vi "Piezo_Positioning_MD.vi"() -> ()   [LabVIEW 2012]
uses:
  <vilib>/DAQmx/write.llb/DAQmx Write (Analog DBL 1Chan 1Samp).vi
  GFG/GFGbooleanGet.vi
  <vilib>/DAQmx/create/channels.llb/DAQmx Create Channel (AO-Voltage-Basic).vi
  <vilib>/DAQmx/miscellaneous.llb/DAQmx Fill In Error Info.vi
  GFG/GFGnumericGet.vi
  GFG/GFG library.lvlib
panel:
  in  "Step Size (um)":u16(ring)=5 items=["1"=1, "2"=2, "5"=5, "10"=10, "20"=20, "50"=50, "100"=100]
  in  "Z DOWN":bool
  in  "Z UP":bool
  in  "Z-Spacing (microns)":dbl=1.0 min=0.1
  in  "Clear Stack":bool
  in  "Remove Last":bool
  in  "Add Plane":bool
  out "Configured Stack":dbl[][](array[numeric])
  in  "Z - Piezo Offset  (um)":i32 max=600
  # "X"
  # "Y"
  # "Z"
  # "Laser 1"
  # "Laser 2"
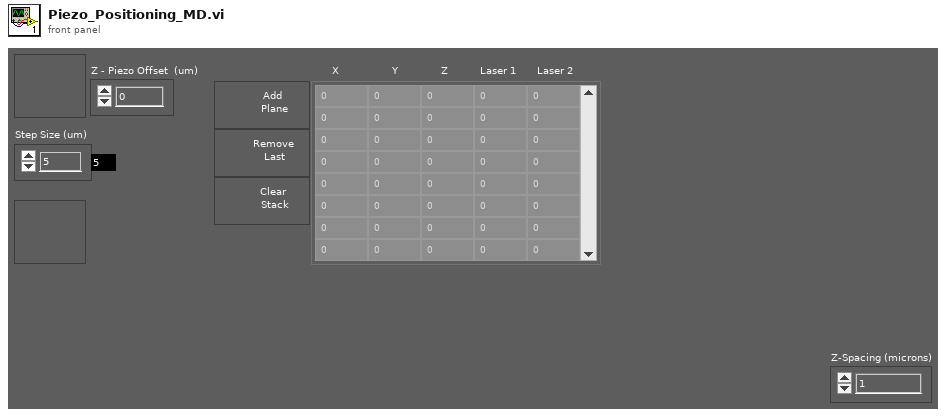
[diagram p1: front panel]
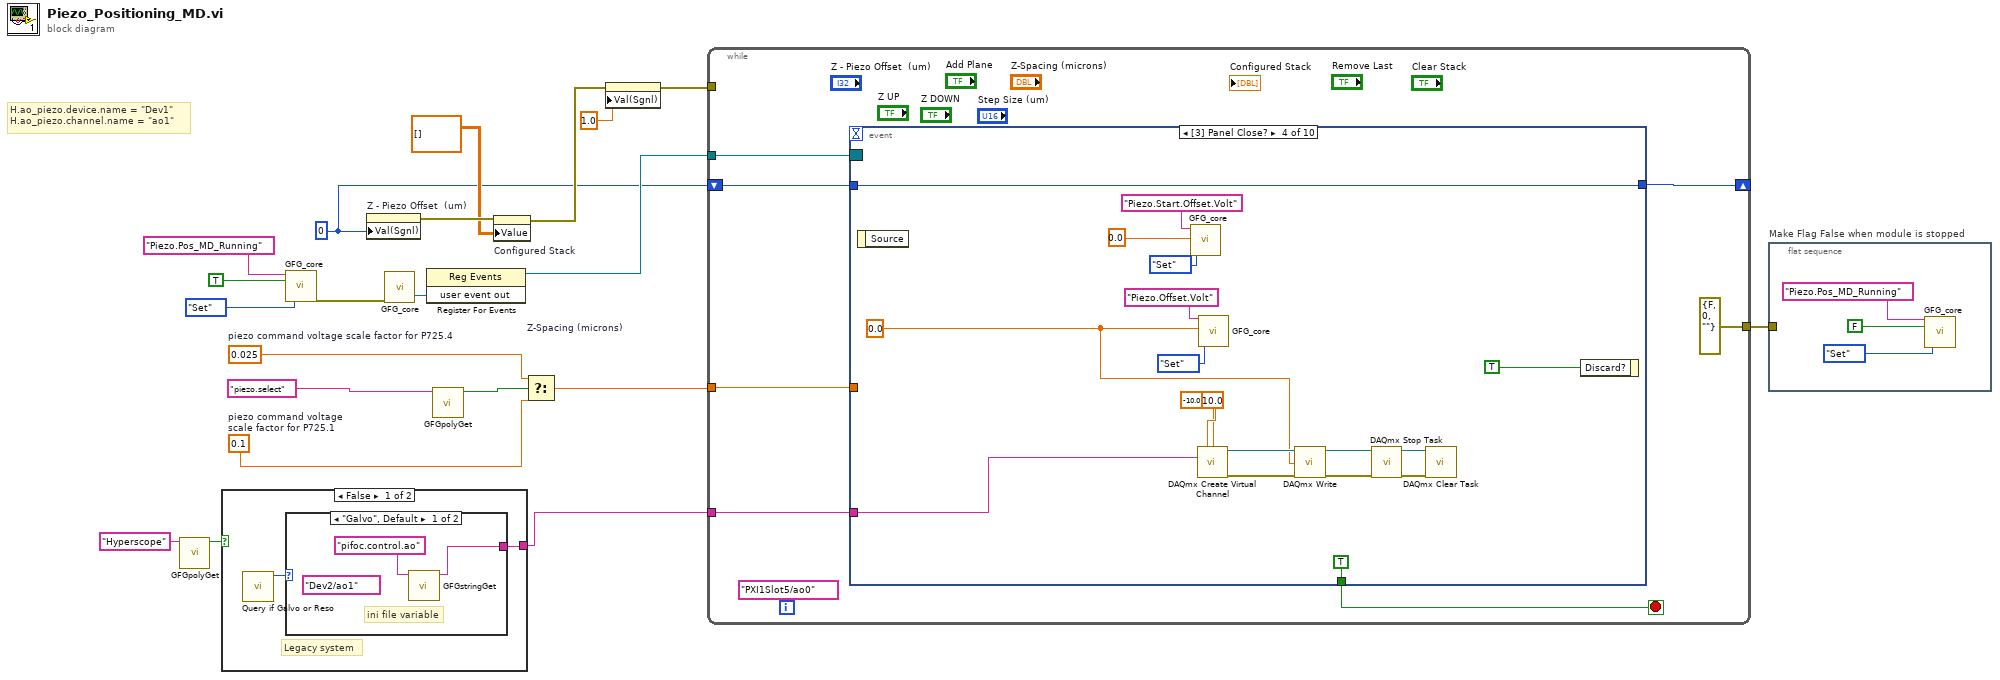
[diagram p0: block diagram]
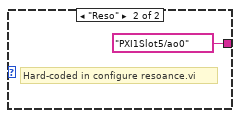
[diagram p2: hidden frame]
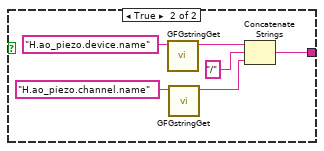
[diagram p3: hidden frame]
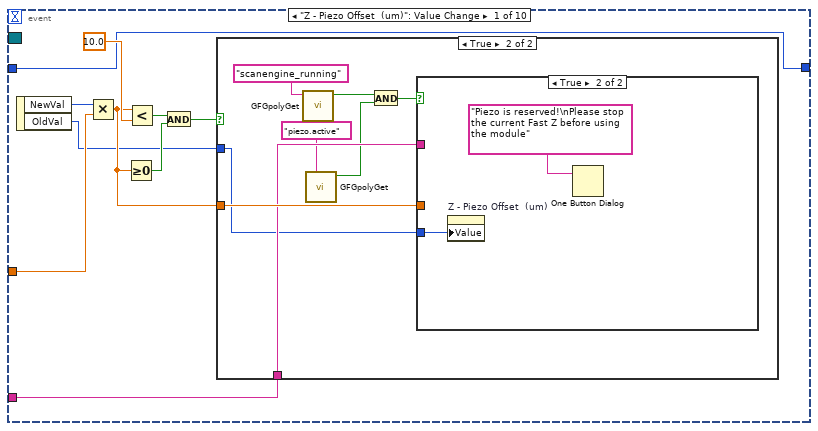
[diagram p4: hidden frame]
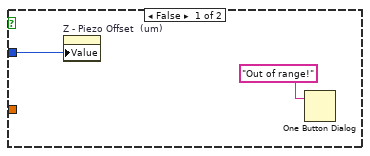
[diagram p5: hidden frame]
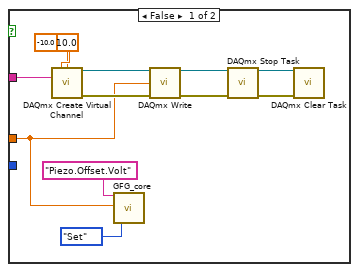
[diagram p6: hidden frame]
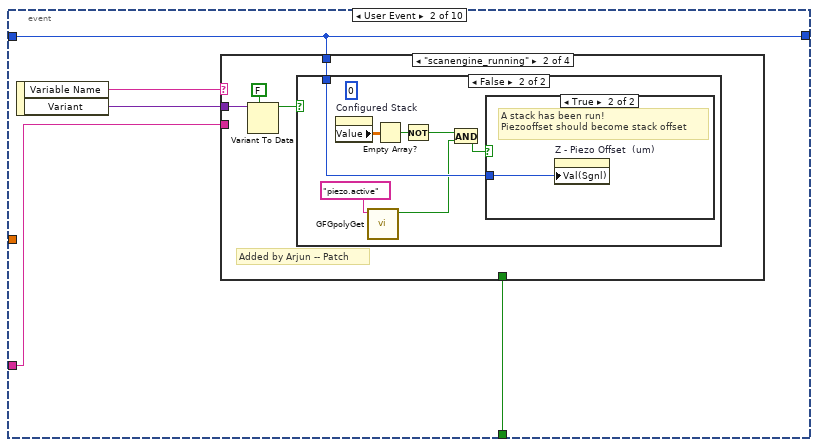
[diagram p7: hidden frame]
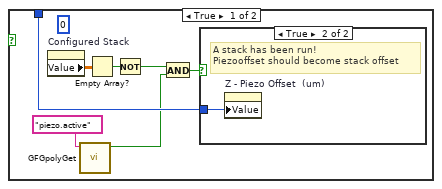
[diagram p9: hidden frame]
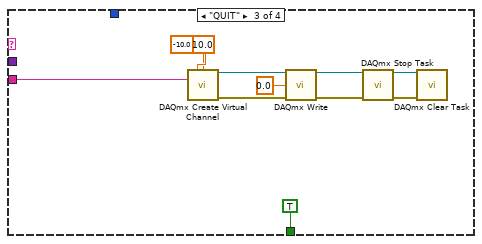
[diagram p12: hidden frame]
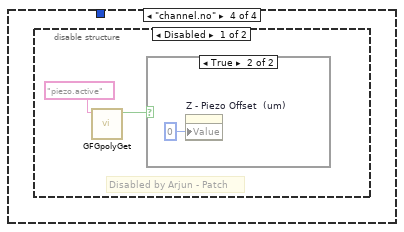
[diagram p13: hidden frame]
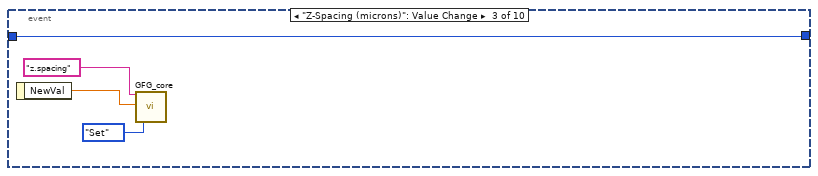
[diagram p16: hidden frame]
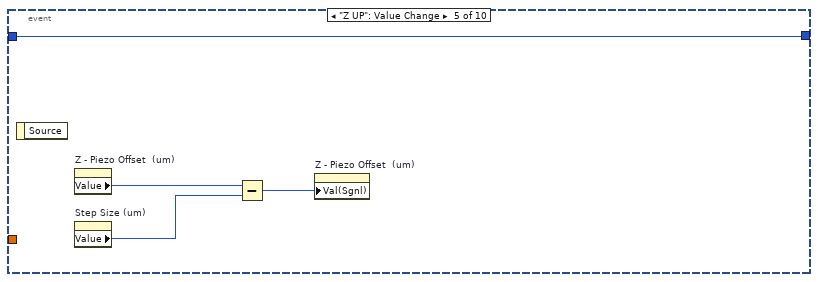
[diagram p17: hidden frame]
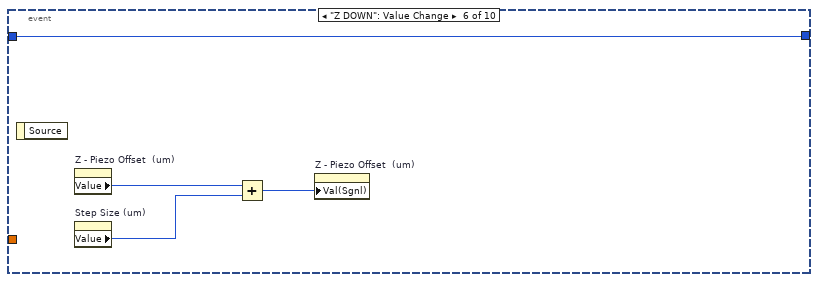
[diagram p18: hidden frame]
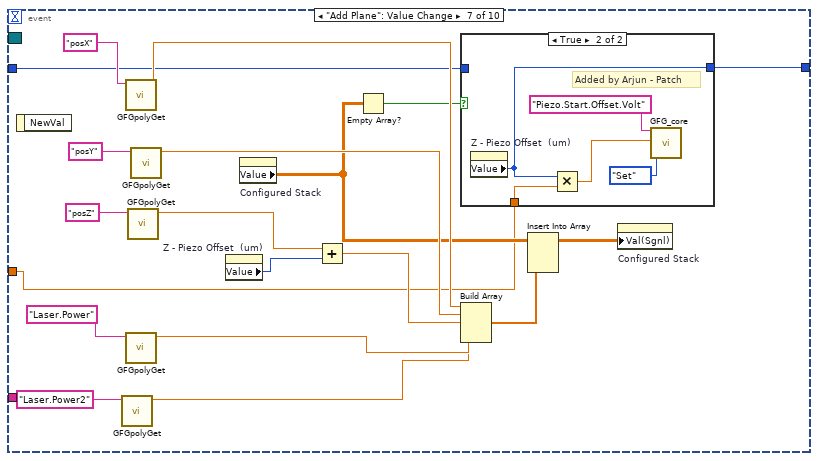
[diagram p19: hidden frame]
diagram:
  w9 = 0 ("Value (Signaling)")
  w18 = 0.1  # piezo command voltage scale factor for P725.1
  w19 = 0.025  # piezo command voltage scale factor for P725.4
  # "H.ao_piezo.device.name = \"Dev1\"\nH.ao_piezo.channel.name = \"ao1\""
  n1 = call-poly "GFGpolyGet.vi"("Variable Name in"="Hyperscope") -> ("Boolean Value OUT"=w2:bool)  [unwired: 9 in, 1 out]
  n2 = case shown="False" w2 {
    tunnel: [w23 w27] -> w1
    frame False {
      # "Legacy system"
      n3 = call "Query if Galvo or Reso.vi"() -> ("System Type"=w22:enum16{"Galvo", "Reso"})  [unwired: 10 in, 1 out]
      n4 = case shown="\"Galvo\", Default" w22 {
        tunnel: [w24 tag "PXI1Slot5/ao0" ("AO Channel for Piezo")] -> w23
        frame "Galvo", Default {
          (unwired) tag "Dev2/ao1" ("AO Channel for Piezo")
          # "ini file variable"
          n5 = call "GFGstringGet.vi"("Variable Name in"="pifoc.control.ao") -> ("String"=w24:string)  [unwired: 9 in, 1 out]
        }
        frame "Reso" {
          # "Hard-coded in configure resoance.vi"
        }
      }
    }
    frame True {
      n6 = call "GFGstringGet.vi"("Variable Name in"="H.ao_piezo.device.name") -> ("String"=w30:string)  [unwired: 9 in, 1 out]
      n7 = call "GFGstringGet.vi"("Variable Name in"="H.ao_piezo.channel.name") -> ("String"=w28:string)  [unwired: 9 in, 1 out]
      n8 = Concatenate Strings(w30, "/" ("string"), w28) -> (w27:string)
    }
  }
  n9 = call "GFG_core.vi"("Variable Name in"="Piezo.Pos_MD_Running", "Variant in"=TRUE, "Action"=enum16{"Init", "Set", "Get", "Clear"}."Set") -> ("error out"=w5:errorcluster)  [unwired: 10 in, 6 out]
  n10 = property on="Z - Piezo Offset  (um)" class="DigNum (strict)"("Val(Sgnl)"=w9) -> (error out=w14:errorcluster)  [unwired: 2 in, 1 out]
  n11 = call "GFG_core.vi"("error in (no error)"=w5) -> ("user event out"=w11:refnum<user-event>)  [unwired: 12 in, 6 out]
  n12 = register-events(w11) -> (reference out=w10:refnum<event-registration>)  [unwired: 2 in, 1 out]
  n13 = call-poly "GFGpolyGet.vi"("Variable Name in"="piezo.select") -> ("Boolean Value OUT"=w16:bool)  [unwired: 9 in, 1 out]
  n14 = property on="Configured Stack" class="Arr (strict)"(error in=w14, "Value"=dbl[][] []) -> (error out=w12:errorcluster)  [unwired: 1 in, 1 out]
  n15 = Select(t=w19, s=w16, f=w18) -> (s? t:f=w15:dbl)
  n16 = property on="Z-Spacing (microns)" class="DigNum (strict)"(error in=w12, "Val(Sgnl)"=1.0 ("Value (Signaling)")) -> (error out=w20:errorcluster)  [unwired: 1 in, 1 out]
  n17 = while {
    tunnel: w20 -> [_]
    tunnel: w15 -> [w38]
    tunnel: w10 -> [w37]
    shift-right: [w36] -> _
    shift-left: w9 -> [w35]
    tunnel: [errorcluster {"status"=FALSE, "code"=0, "source"=""} ("error constant")] -> w4
    tunnel: w1 -> [w33]
    stop <- w39 stop-if-true
    (unwired) tag "PXI1Slot5/ao0" ("AO Channel for Piezo")
    n18 = event shown="[3] Panel Close?" {
      selector: w37 -> [_ _ _ _ _ _ _ _ _ _]
      dyn-events: _ -> [_ _ _ _ _ _ _ _ _ _]
      timeout: _ -> [_ _ _ _ _ _ _ _ _ _]
      tunnel: [_ w77 _ TRUE _ _ _ _ _ _] -> w39
      tunnel: w38 -> [w44 _ _ _ _ _ w145 w170 w184 _]
      tunnel: w33 -> [w41 w75 _ w119 _ _ _ _ _ _]
      tunnel: [w40 w74 w113 w117 w135 w139 w144 w168 w181 w191] -> w36
      tunnel: w35 -> [w40 w74 w113 w117 w135 w139 w143 w169 _ w191]
      event "Z - Piezo Offset  (um)": Value Change {
        n19 = event-data() -> ("NewVal"=w49:i32, "OldVal"=w42:i32)  [unwired: 1 in]
        n20 = Multiply(x=w49, y=w44) -> (x*y=w43:dbl)
        n21 = Greater Or Equal To 0?(x=w43) -> (x >= 0?=w45:bool)
        n22 = Less?(x=w43, y=10.0) -> (x < y?=w48:bool)
        n23 = And(x=w48, y=w45) -> (x .and. y?=w46:bool)
        n24 = case shown="True" w46 {
          tunnel: w43 -> [_ w59]
          tunnel: w42 -> [w50 w52]
          tunnel: w41 -> [_ w58]
          frame False {
            n25 = property on="Z - Piezo Offset  (um)" class="DigNum (strict)"("Value"=w50) -> ()  [unwired: 2 in, 2 out]
            n26 = One Button Dialog(message="Out of range!") -> ()  [unwired: 1 in, 1 out]
          }
          frame True {
            n27 = call-poly "GFGpolyGet.vi"("Variable Name in"="scanengine_running") -> ("Boolean Value OUT"=w55:bool)  [unwired: 9 in, 1 out]
            n28 = call-poly "GFGpolyGet.vi"("Variable Name in"="piezo.active") -> ("Boolean Value OUT"=w54:bool)  [unwired: 9 in, 1 out]
            n29 = And(x=w55, y=w54) -> (x .and. y?=w53:bool)
            n30 = case shown="True" w53 {
              tunnel: w59 -> [w61 _]
              tunnel: w58 -> [w60 _]
              tunnel: w52 -> [_ w72]
              frame False {
                n31 = call-poly <vilib>:"DAQmx Create Virtual Channel.vi"("maximum value"=10.0, "minimum value"=-10.0, "physical channels"=w60) -> ("task out"=w69:refnum<k21>, "error out"=w65:errorcluster)  [unwired: 11 in]
                n32 = call "GFG_core.vi"("Variable Name in"="Piezo.Offset.Volt", "Variant in"=w61, "Action"=enum16{"Init", "Set", "Get", "Clear"}."Set") -> ()  [unwired: 10 in, 7 out]
                n33 = call-poly <vilib>:"DAQmx Write.vi"("task/channels in"=w69, "data"=w61, "error in"=w65) -> ("task out"=w66:refnum<k21>, "error out"=w64:errorcluster)  [unwired: 10 in, 1 out]
                n34 = call <vilib>:"DAQmx Stop Task.vi"("task/channels in"=w66, "error in"=w64) -> ("task out"=w67:refnum<k21>, "error out"=w68:errorcluster)  [unwired: 12 in]
                n35 = call <vilib>:"DAQmx Clear Task.vi"("task in"=w67, "error in"=w68) -> ()  [unwired: 13 in, 1 out]
              }
              frame True {
                n36 = property on="Z - Piezo Offset  (um)" class="DigNum (strict)"("Value"=w72) -> ()  [unwired: 2 in, 2 out]
                n37 = One Button Dialog(message="Piezo is reserved!\nPlease stop the current Fast Z before using the module") -> ()  [unwired: 1 in, 1 out]
              }
            }
          }
        }
      }
      event User Event {
        n38 = event-data() -> ("Variable Name"=w78:string, "Variant"=w76:variant)  [unwired: 1 in]
        n39 = case shown="\"scanengine_running\"" w78 {
          tunnel: [_ _ TRUE _] -> w77
          tunnel: w76 -> [_ w82 _ _]
          tunnel: w75 -> [_ _ w100 _]
          tunnel: w74 -> [_ w79 _ _]
          frame "False", Default {
          }
          frame "scanengine_running" {
            # "Added by Arjun -- Patch"
            n40 = Variant To Data(type=FALSE, Variant=w82) -> (data=w80:bool)  [unwired: 1 in, 1 out]
            n41 = case shown="False" w80 {
              tunnel: w79 -> [w89 w97]
              frame True {
                (unwired) 0 ("Z - Piezo Offset  (um)")
                n42 = property on="Configured Stack" class="Arr (strict)"() -> ("Value"=w88:dbl[][])  [unwired: 2 in, 2 out]
                n43 = call-poly "GFGpolyGet.vi"("Variable Name in"="piezo.active") -> ("Boolean Value OUT"=w84:bool)  [unwired: 9 in, 1 out]
                n44 = Empty Array?(array=w88) -> (empty?=w87:bool)
                n45 = Not(x=w87) -> (.not. x?=w83:bool)
                n46 = And(x=w83, y=w84) -> (x .and. y?=w85:bool)
                n47 = case shown="True" w85 {
                  tunnel: w89 -> [_ w90]
                  frame False {
                  }
                  frame True {
                    # "A stack has been run!\nPiezooffset should become stack offset"
                    n48 = property on="Z - Piezo Offset  (um)" class="DigNum (strict)"("Value"=w90) -> ()  [unwired: 2 in, 2 out]
                  }
                }
              }
              frame False {
                (unwired) 0 ("Z - Piezo Offset  (um)")
                n49 = property on="Configured Stack" class="Arr (strict)"() -> ("Value"=w96:dbl[][])  [unwired: 2 in, 2 out]
                n50 = call-poly "GFGpolyGet.vi"("Variable Name in"="piezo.active") -> ("Boolean Value OUT"=w93:bool)  [unwired: 9 in, 1 out]
                n51 = Empty Array?(array=w96) -> (empty?=w95:bool)
                n52 = Not(x=w95) -> (.not. x?=w92:bool)
                n53 = And(x=w92, y=w93) -> (x .and. y?=w91:bool)
                n54 = case shown="True" w91 {
                  tunnel: w97 -> [_ w98]
                  frame False {
                  }
                  frame True {
                    # "A stack has been run!\nPiezooffset should become stack offset"
                    n55 = property on="Z - Piezo Offset  (um)" class="DigNum (strict)"("Val(Sgnl)"=w98) -> ()  [unwired: 2 in, 2 out]
                  }
                }
              }
            }
          }
          frame "QUIT" {
            n56 = call-poly <vilib>:"DAQmx Create Virtual Channel.vi"("maximum value"=10.0, "minimum value"=-10.0, "physical channels"=w100) -> ("task out"=w106:refnum<k21>, "error out"=w102:errorcluster)  [unwired: 11 in]
            n57 = call-poly <vilib>:"DAQmx Write.vi"("task/channels in"=w106, "data"=0.0 ("maximum value"), "error in"=w102) -> ("task out"=w103:refnum<k21>, "error out"=w101:errorcluster)  [unwired: 10 in, 1 out]
            n58 = call <vilib>:"DAQmx Stop Task.vi"("task/channels in"=w103, "error in"=w101) -> ("task out"=w104:refnum<k21>, "error out"=w105:errorcluster)  [unwired: 12 in]
            n59 = call <vilib>:"DAQmx Clear Task.vi"("task in"=w104, "error in"=w105) -> ()  [unwired: 13 in, 1 out]
          }
          frame "channel.no" {
            n60 = disable-structure shown="Disabled" {
              frame Disabled {
                # "Disabled by Arjun - Patch"
                n61 = call-poly "GFGpolyGet.vi"("Variable Name in"="piezo.active") -> ("Boolean Value OUT"=w110:bool)  [unwired: 9 in, 1 out]
                n62 = case shown="True" w110 {
                  frame False {
                  }
                  frame True {
                    n63 = property on="Z - Piezo Offset  (um)" class="DigNum (strict)"("Value"=0 ("Z - Piezo Offset  (um)")) -> ()  [unwired: 2 in, 2 out]
                  }
                }
              }
              frame Enabled {
              }
            }
          }
        }
      }
      event "Z-Spacing (microns)": Value Change {
        n64 = event-data() -> ("NewVal"=w114:dbl)  [unwired: 1 in]
        n65 = call "GFG_core.vi"("Variable Name in"="z.spacing", "Variant in"=w114, "Action"=enum16{"Init", "Set", "Get", "Clear"}."Set") -> ()  [unwired: 10 in, 7 out]
      }
      event Panel Close? {
        w118 = 0.0 ("Value (Signaling)")
        n66 = event-data() -> ()  [unwired: 1 in, 1 out]
        n67 = call "GFG_core.vi"("Variable Name in"="Piezo.Start.Offset.Volt", "Variant in"=0.0 ("Value (Signaling)"), "Action"=enum16{"Init", "Set", "Get", "Clear"}."Set") -> ()  [unwired: 10 in, 7 out]
        n68 = call-poly <vilib>:"DAQmx Create Virtual Channel.vi"("maximum value"=10.0, "minimum value"=-10.0, "physical channels"=w119) -> ("task out"=w125:refnum<k21>, "error out"=w121:errorcluster)  [unwired: 11 in]
        n69 = call "GFG_core.vi"("Variable Name in"="Piezo.Offset.Volt", "Variant in"=w118, "Action"=enum16{"Init", "Set", "Get", "Clear"}."Set") -> ()  [unwired: 10 in, 7 out]
        n70 = call-poly <vilib>:"DAQmx Write.vi"("task/channels in"=w125, "data"=w118, "error in"=w121) -> ("task out"=w122:refnum<k21>, "error out"=w120:errorcluster)  [unwired: 10 in, 1 out]
        n71 = call <vilib>:"DAQmx Stop Task.vi"("task/channels in"=w122, "error in"=w120) -> ("task out"=w123:refnum<k21>, "error out"=w124:errorcluster)  [unwired: 12 in]
        n72 = call <vilib>:"DAQmx Clear Task.vi"("task in"=w123, "error in"=w124) -> ()  [unwired: 13 in, 1 out]
        n73 = event-data("Discard?"=TRUE) -> ()  [unwired: 1 in, 1 out]
      }
      event "Z UP": Value Change {
        n74 = event-data() -> ()  [unwired: 1 in, 1 out]
        n75 = property on="Z - Piezo Offset  (um)" class="DigNum (strict)"() -> ("Value"=w138:i32)  [unwired: 2 in, 2 out]
        n76 = property on="Step Size (um)" class="Ring (strict)"() -> ("Value"=w137:u16)  [unwired: 2 in, 2 out]
        n77 = Subtract(x=w138, y=w137) -> (x-y=w136:i32)
        n78 = property on="Z - Piezo Offset  (um)" class="DigNum (strict)"("Val(Sgnl)"=w136) -> ()  [unwired: 2 in, 2 out]
      }
      event "Z DOWN": Value Change {
        n79 = event-data() -> ()  [unwired: 1 in, 1 out]
        n80 = property on="Z - Piezo Offset  (um)" class="DigNum (strict)"() -> ("Value"=w142:i32)  [unwired: 2 in, 2 out]
        n81 = property on="Step Size (um)" class="Ring (strict)"() -> ("Value"=w141:u16)  [unwired: 2 in, 2 out]
        n82 = Add(x=w142, y=w141) -> (x+y=w140:i32)
        n83 = property on="Z - Piezo Offset  (um)" class="DigNum (strict)"("Val(Sgnl)"=w140) -> ()  [unwired: 2 in, 2 out]
      }
      event "Add Plane": Value Change {
        n84 = event-data() -> ()  [unwired: 1 in, 1 out]
        n85 = call-poly "GFGpolyGet.vi"("Variable Name in"="Laser.Power2") -> ("Numeric"=w149:dbl)  [unwired: 8 in, 2 out]
        n86 = call-poly "GFGpolyGet.vi"("Variable Name in"="posX") -> ("Numeric"=w156:dbl)  [unwired: 8 in, 2 out]
        n87 = call-poly "GFGpolyGet.vi"("Variable Name in"="Laser.Power") -> ("Numeric"=w150:dbl)  [unwired: 8 in, 2 out]
        n88 = call-poly "GFGpolyGet.vi"("Variable Name in"="posZ") -> ("Numeric"=w157:dbl)  [unwired: 8 in, 2 out]
        n89 = call-poly "GFGpolyGet.vi"("Variable Name in"="posY") -> ("Numeric"=w155:dbl)  [unwired: 8 in, 2 out]
        n90 = property on="Z - Piezo Offset  (um)" class="DigNum (strict)"() -> ("Value"=w158:i32)  [unwired: 2 in, 2 out]
        n91 = property on="Configured Stack" class="Arr (strict)"() -> ("Value"=w147:dbl[][])  [unwired: 2 in, 2 out]
        n92 = Add(x=w157, y=w158) -> (x+y=w154:dbl)
        n93 = Empty Array?(array=w147) -> (empty?=w146:bool)
        n94 = case shown="True" w146 {
          tunnel: w145 -> [_ w165]
          tunnel: [w162 w163] -> w144
          tunnel: w143 -> [w162 _]
          frame False {
          }
          frame True {
            # "Added by Arjun - Patch"
            n95 = property on="Z - Piezo Offset  (um)" class="DigNum (strict)"() -> ("Value"=w163:i32)  [unwired: 2 in, 2 out]
            n96 = Multiply(x=w163, y=w165) -> (x*y=w164:dbl)
            n97 = call "GFG_core.vi"("Variable Name in"="Piezo.Start.Offset.Volt", "Variant in"=w164, "Action"=enum16{"Init", "Set", "Get", "Clear"}."Set") -> ()  [unwired: 10 in, 7 out]
          }
        }
        n98 = Build Array(w156, w155, w154, w150, w149) -> (w153:dbl[])
        n99 = Insert Into Array(array=w147, new element=w153) -> (w148:dbl[][])  [unwired: 2 in]
        n100 = property on="Configured Stack" class="Arr (strict)"("Val(Sgnl)"=w148) -> ()  [unwired: 2 in, 2 out]
      }
      event "Remove Last": Value Change {
        n101 = event-data() -> ()  [unwired: 1 in, 1 out]
        n102 = property on="Configured Stack" class="Arr (strict)"() -> ("Value"=w171:dbl[][])  [unwired: 2 in, 2 out]
        n103 = Empty Array?(array=w171) -> (empty?=w172:bool)
        n104 = case shown="True" w172 {
          tunnel: w170 -> [_ w176]
          tunnel: w169 -> [w174 _]
          tunnel: [w174 w175] -> w168
          frame False {
          }
          frame True {
            w178 = 0.0  # Stack start voltage
            # "Added by Arjun - Patch"
            n105 = Divide(x=w178, y=w176) -> (x/y=w177:dbl)
            n106 = To Long Integer(number=w177) -> (32bit integer=w175:i32)
            n107 = call "GFG_core.vi"("Variable Name in"="Piezo.Start.Offset.Volt", "Variant in"=w178, "Action"=enum16{"Init", "Set", "Get", "Clear"}."Set") -> ()  [unwired: 10 in, 7 out]
          }
        }
        n108 = Delete From Array(array=w171) -> (array with subset deleted=w173:dbl[][])  [unwired: 3 in, 1 out]
        n109 = property on="Configured Stack" class="Arr (strict)"("Val(Sgnl)"=w173) -> ()  [unwired: 2 in, 2 out]
      }
      event "Clear Stack": Value Change {
        w183 = 0.0  # Stack start voltage
        # "Added by Arjun - Patch"
        n110 = event-data() -> ()  [unwired: 1 in, 1 out]
        n111 = property on="Configured Stack" class="Arr (strict)"("Val(Sgnl)"=dbl[][] [] ("Value (Signaling)")) -> ()  [unwired: 2 in, 2 out]
        n112 = call "GFG_core.vi"("Variable Name in"="clear all", "Variant in"=TRUE, "Action"=enum16{"Init", "Set", "Get", "Clear"}."Set") -> ()  [unwired: 10 in, 7 out]
        n113 = call "GFG_core.vi"("Variable Name in"="Piezo.Start.Offset.Volt", "Variant in"=w183, "Action"=enum16{"Init", "Set", "Get", "Clear"}."Set") -> ()  [unwired: 10 in, 7 out]
        n114 = Divide(x=w183, y=w184) -> (x/y=w182:dbl)
        n115 = To Long Integer(number=w182) -> (32bit integer=w181:i32)
      }
      event "Configured Stack": Value Change {
        n116 = event-data() -> ("NewVal"=w192:dbl[][])  [unwired: 1 in]
        n117 = call "GFG_core.vi"("Variable Name in"="pos  pockels cell PMT Data", "Variant in"=w192, "Action"=enum16{"Init", "Set", "Get", "Clear"}."Set") -> ()  [unwired: 10 in, 7 out]
      }
    }
  }
  n118 = flat-sequence "Make Flag False when module is stopped" {
    tunnel: w4 -> [_]
    frame #0 {
      n119 = call "GFG_core.vi"("Variable Name in"="Piezo.Pos_MD_Running", "Variant in"=FALSE, "Action"=enum16{"Init", "Set", "Get", "Clear"}."Set") -> ()  [unwired: 10 in, 7 out]
    }
  }
